vi "get arm refnums.vi"(8 "error in (no error)":errorcluster, 11 "Elevator Concrete in":refnum<class "Elevator Concrete.lvclass">) -> (0 "error out":errorcluster, 1 "motor refnums":T1, 3 "Elevator Concrete out":refnum<class "Elevator Concrete.lvclass">)   [LabVIEW 2018, in "Elevator.lvlib" / "Elevator Concrete.lvclass"]
uses:
  Elevator Concrete.lvclass
  Elevator Concrete.lvclass/Elevator Concrete.ctl
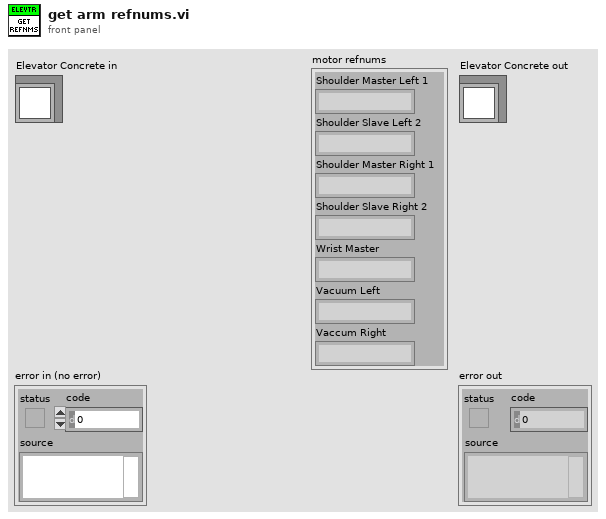
[diagram p1: front panel]
types:
  T1 = cluster{"Shoulder Master Left 1":string, "Shoulder Slave Left 2":string, "Shoulder Master Right 1":string, "Shoulder Slave Right 2 ":string, "Wrist Master ":string, "Vacuum Left":string, "Vaccum Right":string}
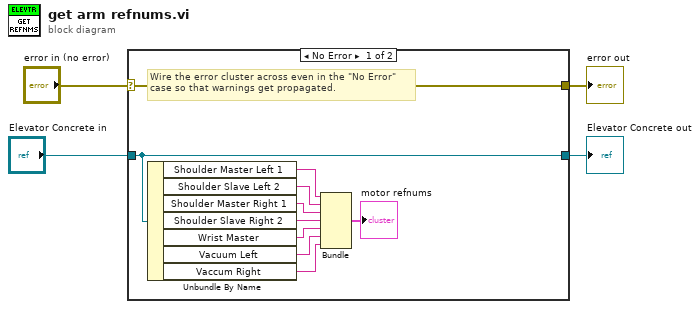
[diagram p0: block diagram]
diagram:
  n1 = case shown="No Error" "error in (no error)" {
    selector: "error in (no error)" -> [w14 w16]
    tunnel: [w14 w16] -> w3
    tunnel: [w13 w15] -> w1
    tunnel: "Elevator Concrete in" -> [w13 w15]
    frame No Error {
      # "Wire the error cluster across even in the \"No Error\"\ncase so that warnings get propagated."
      n2 = Unbundle By Name(w13) -> ("Shoulder Master Left 1"=w12:string, "Shoulder Slave Left 2"=w11:string, "Shoulder Master Right 1"=w10:string, "Shoulder Slave Right 2"=w9:string, "Wrist Master"=w8:string, "Vacuum Left"=w7:string, "Vaccum Right"=w6:string)
      n3 = Bundle("Shoulder Master Left 1"=w12, "Shoulder Slave Left 2"=w11, "Shoulder Master Right 1"=w10, "Shoulder Slave Right 2"=w9, "Wrist Master"=w8, "Vacuum Left"=w7, "Vaccum Right"=w6) -> (→"motor refnums":T1)  [unwired: 1 in]
    }
    frame Error {
    }
  }
  "error out" <- w3
  "Elevator Concrete out" <- w1
